vi "CheckForErrorsFloat.vi"(5 "Maximum":dbl, 7 "Minimum":dbl, 10 "Parameter Index":i32, 11 "Parameters":string[](array[string])) -> (0 "Error":errorcluster, 3 "Output":dbl)   [LabVIEW 2019]
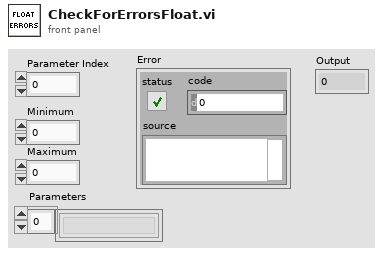
[diagram p1: front panel]
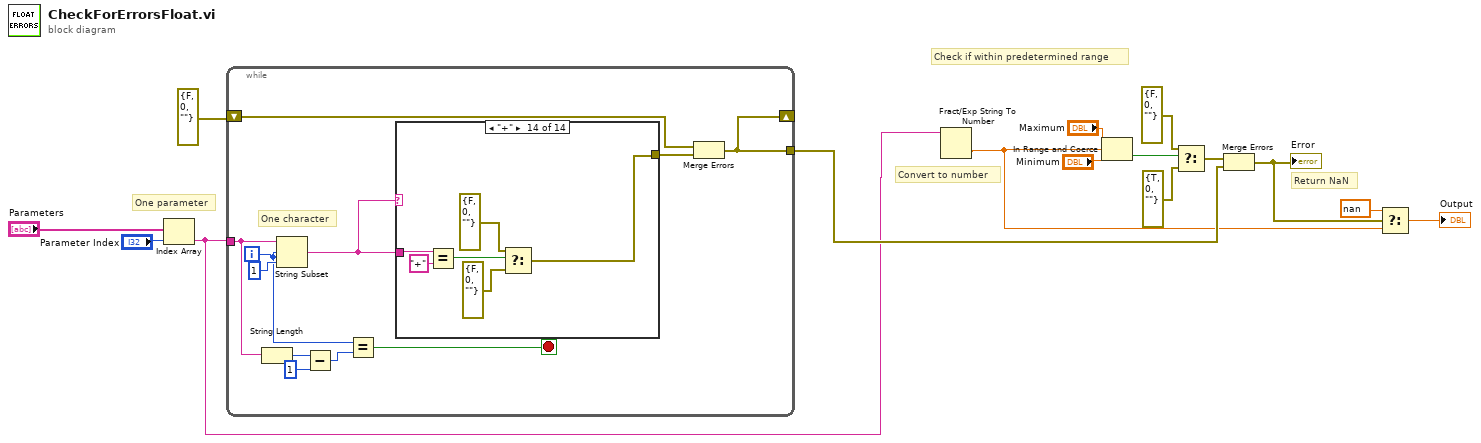
[diagram p0: block diagram]
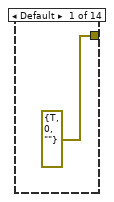
[diagram p2: hidden frame]
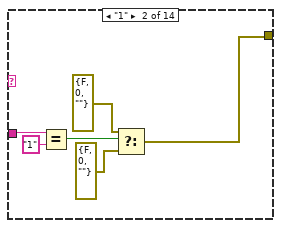
[diagram p3: hidden frame]
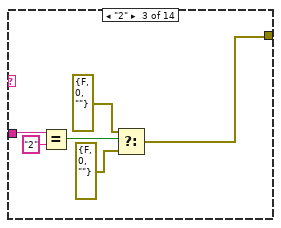
[diagram p4: hidden frame]
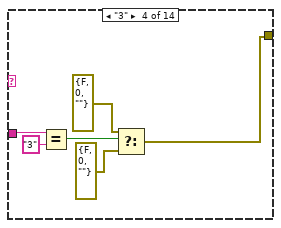
[diagram p5: hidden frame]
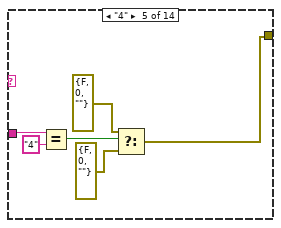
[diagram p6: hidden frame]
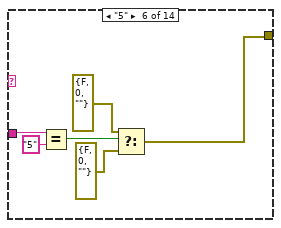
[diagram p7: hidden frame]
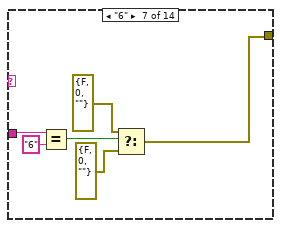
[diagram p8: hidden frame]
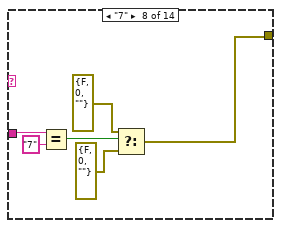
[diagram p9: hidden frame]
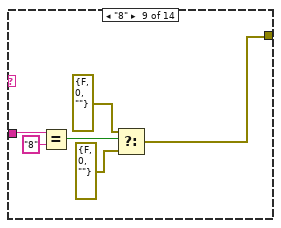
[diagram p10: hidden frame]
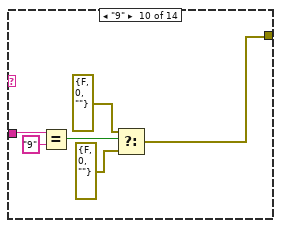
[diagram p11: hidden frame]
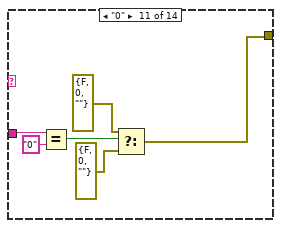
[diagram p12: hidden frame]
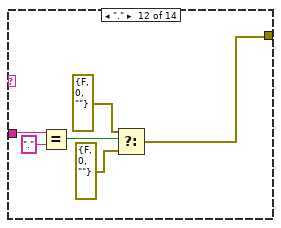
[diagram p13: hidden frame]
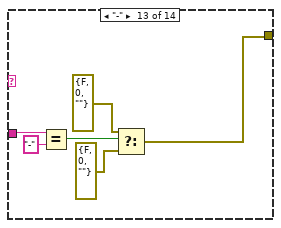
[diagram p14: hidden frame]
diagram:
  # "Convert to number"
  # "Return NaN"
  # "Check if within predetermined range"
  # "One parameter"
  n1 = Index Array(array="Parameters", index="Parameter Index") -> (element=w5:string)
  n2 = while {
    tunnel: w5 -> [w25]
    shift-right: [w16] -> _
    shift-left: errorcluster {"status"=FALSE, "code"=0, "source"=""} ("error constant") -> [w17]
    tunnel: [w16] -> w7
    i -> [w22]
    stop <- w24 stop-if-true
    # "One character"
    n3 = String Length(string=w25) -> (length=w21:i32)
    n4 = String Subset(string=w25, offset (0)=w22, length (rest)=1) -> (substring=w23:string)
    n5 = Subtract(x=w21, y=1) -> (x-y=w19:i32)
    n6 = Equal?(x=w22, y=w19) -> (x = y?=w24:bool)
    n7 = case shown="\"+\"" w23 {
      tunnel: w23 -> [_ w31 w37 w43 w49 w55 w61 w67 w73 w79 w85 w91 w97 w103]
      tunnel: [errorcluster {"status"=TRUE, "code"=0, "source"=""} ("error constant") w28 w34 w40 w46 w52 w58 w64 w70 w76 w82 w88 w94 w100] -> w18
      frame Default {
      }
      frame "1" {
        n8 = Equal?(x=w31, y="1") -> (x = y?=w32:bool)
        n9 = Select(t=errorcluster {"status"=FALSE, "code"=0, "source"=""} ("error constant"), s=w32, f=errorcluster {"status"=FALSE, "code"=0, "source"=""} ("error constant")) -> (s? t:f=w28:errorcluster)
      }
      frame "2" {
        n10 = Equal?(x=w37, y="2") -> (x = y?=w38:bool)
        n11 = Select(t=errorcluster {"status"=FALSE, "code"=0, "source"=""} ("error constant"), s=w38, f=errorcluster {"status"=FALSE, "code"=0, "source"=""} ("error constant")) -> (s? t:f=w34:errorcluster)
      }
      frame "3" {
        n12 = Equal?(x=w43, y="3") -> (x = y?=w44:bool)
        n13 = Select(t=errorcluster {"status"=FALSE, "code"=0, "source"=""} ("error constant"), s=w44, f=errorcluster {"status"=FALSE, "code"=0, "source"=""} ("error constant")) -> (s? t:f=w40:errorcluster)
      }
      frame "4" {
        n14 = Equal?(x=w49, y="4") -> (x = y?=w50:bool)
        n15 = Select(t=errorcluster {"status"=FALSE, "code"=0, "source"=""} ("error constant"), s=w50, f=errorcluster {"status"=FALSE, "code"=0, "source"=""} ("error constant")) -> (s? t:f=w46:errorcluster)
      }
      frame "5" {
        n16 = Equal?(x=w55, y="5") -> (x = y?=w56:bool)
        n17 = Select(t=errorcluster {"status"=FALSE, "code"=0, "source"=""} ("error constant"), s=w56, f=errorcluster {"status"=FALSE, "code"=0, "source"=""} ("error constant")) -> (s? t:f=w52:errorcluster)
      }
      frame "6" {
        n18 = Equal?(x=w61, y="6") -> (x = y?=w62:bool)
        n19 = Select(t=errorcluster {"status"=FALSE, "code"=0, "source"=""} ("error constant"), s=w62, f=errorcluster {"status"=FALSE, "code"=0, "source"=""} ("error constant")) -> (s? t:f=w58:errorcluster)
      }
      frame "7" {
        n20 = Equal?(x=w67, y="7") -> (x = y?=w68:bool)
        n21 = Select(t=errorcluster {"status"=FALSE, "code"=0, "source"=""} ("error constant"), s=w68, f=errorcluster {"status"=FALSE, "code"=0, "source"=""} ("error constant")) -> (s? t:f=w64:errorcluster)
      }
      frame "8" {
        n22 = Equal?(x=w73, y="8") -> (x = y?=w74:bool)
        n23 = Select(t=errorcluster {"status"=FALSE, "code"=0, "source"=""} ("error constant"), s=w74, f=errorcluster {"status"=FALSE, "code"=0, "source"=""} ("error constant")) -> (s? t:f=w70:errorcluster)
      }
      frame "9" {
        n24 = Equal?(x=w79, y="9") -> (x = y?=w80:bool)
        n25 = Select(t=errorcluster {"status"=FALSE, "code"=0, "source"=""} ("error constant"), s=w80, f=errorcluster {"status"=FALSE, "code"=0, "source"=""} ("error constant")) -> (s? t:f=w76:errorcluster)
      }
      frame "0" {
        n26 = Equal?(x=w85, y="0") -> (x = y?=w86:bool)
        n27 = Select(t=errorcluster {"status"=FALSE, "code"=0, "source"=""} ("error constant"), s=w86, f=errorcluster {"status"=FALSE, "code"=0, "source"=""} ("error constant")) -> (s? t:f=w82:errorcluster)
      }
      frame "." {
        n28 = Equal?(x=w91, y=".") -> (x = y?=w92:bool)
        n29 = Select(t=errorcluster {"status"=FALSE, "code"=0, "source"=""} ("error constant"), s=w92, f=errorcluster {"status"=FALSE, "code"=0, "source"=""} ("error constant")) -> (s? t:f=w88:errorcluster)
      }
      frame "-" {
        n30 = Equal?(x=w97, y="-") -> (x = y?=w98:bool)
        n31 = Select(t=errorcluster {"status"=FALSE, "code"=0, "source"=""} ("error constant"), s=w98, f=errorcluster {"status"=FALSE, "code"=0, "source"=""} ("error constant")) -> (s? t:f=w94:errorcluster)
      }
      frame "+" {
        n32 = Equal?(x=w103, y="+") -> (x = y?=w104:bool)
        n33 = Select(t=errorcluster {"status"=FALSE, "code"=0, "source"=""} ("error constant"), s=w104, f=errorcluster {"status"=FALSE, "code"=0, "source"=""} ("error constant")) -> (s? t:f=w100:errorcluster)
      }
    }
    n34 = Merge Errors(w17, w18) -> (w16:errorcluster)
  }
  n35 = Fract/Exp String To Number(string=w5) -> (number=w3:dbl)  [unwired: 3 in, 1 out]
  n36 = In Range and Coerce(upper limit="Maximum", x=w3, lower limit="Minimum") -> (In Range?=w11:bool)  [unwired: 1 out]
  n37 = Select(t=errorcluster {"status"=FALSE, "code"=0, "source"=""} ("error constant"), s=w11, f=errorcluster {"status"=TRUE, "code"=0, "source"=""} ("error constant")) -> (s? t:f=w8:errorcluster)
  n38 = Merge Errors(w8, w7) -> (w4:errorcluster)
  "Error" <- w4
  n39 = Select(t=nan, s=w4, f=w3) -> (s? t:f=→"Output":dbl)
